vi "Average Sectors.vi"(11 "Preanalysis Stage":bool) -> ()   [LabVIEW 2013]
uses:
  Globals/Accumulated Sector Intensity.vi
  <vilib>/rvi/Memory/Memory_Emulation/nirvimemoryFastEmulationFpgaImpl.vi
  <instcachedir>/0/nirvimemoryFastEmulationFpgaImpl_5FBAB50466BC4C939F684F8805638BFC.lvgen/nirvimemoryFastEmulationFpgaImpl_5FBAB50466BC4C939F684F8805638BFC_001.vi
  <vilib>/rvi/DataTransferAndStorage/Container/Common/niFpgaContainerGetUniqueNameForEmu.vi
  <vilib>/rvi/Memory/Memory_Emulation/nirvimemoryFastEmulation.vi
  <vilib>/rvi/Memory/Memory_Emulation/nirvimemoryEmulation.vi
  Globals/Sector Parameter Global.vi
  <vilib>/rvi/FIFO/Fifo_Resource/nirvififoEmulationWriteFpgaImpl.vi
  <vilib>/rvi/DataTransferAndStorage/Container/XNode/niFpgaContainer.xnode
  <vilib>/rvi/FIFO/Fifo_Resource/nirvififoEmulationWrite.vi
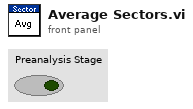
[diagram p1: front panel]
types:
  T1 = cluster{"Accumulated Intensity":fxp<+,20,20>, "Count":fxp<+,12,12>}[]
  T2 = cluster{"Accumulated Intensity":fxp<+,20,20>, "Count":fxp<+,12,12>}
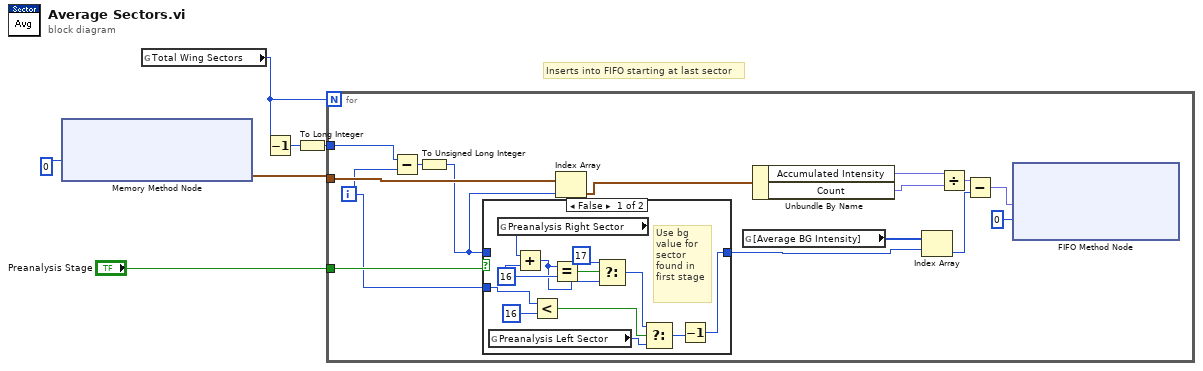
[diagram p0: block diagram]
diagram:
  # "Inserts into FIFO starting at last sector"
  n1 = xnode ("Memory Method Node")("Address"=u32 0) -> ("Data"=w2:T1)  [unwired: 1 in, 1 out]
  n2 = global read "Accumulated Sector Intensity.vi" "Total Wing Sectors"() -> (w4:u8)
  n3 = Decrement(x=w4) -> (x-1=w6:u8)
  n4 = To Long Integer(number=w6) -> (32bit integer=w5:i32)
  n5 = for {
    N: w4 -> [_]
    tunnel: w5 -> [w16]
    tunnel: w2 -> [w14]
    tunnel: "Preanalysis Stage" -> [w10]
    i -> [w7]
    n6 = Subtract(x=w16, y=w7) -> (x-y=w15:i32)
    n7 = To Unsigned Long Integer(number=w15) -> (unsigned 32bit integer=w8:u32)
    n8 = case shown="False" w10 {
      tunnel: [w28 w34] -> w9
      tunnel: w8 -> [_ w34]
      tunnel: w7 -> [w33 _]
      frame False {
        w26 = u8 16 ("y")
        # "Use bg value for sector found in first stage"
        n9 = global read "Sector Parameter Global.vi" "Preanalysis Left Sector"() -> (w30:u8)
        n10 = global read "Sector Parameter Global.vi" "Preanalysis Right Sector"() -> (w23:u8)
        n11 = Add(x=w23, y=w26) -> (x+y=w24:u8)
        n12 = Less?(x=w33, y=16) -> (x < y?=w31:bool)
        n13 = Equal?(x=w24, y=w26) -> (x = y?=w27:bool)
        n14 = Select(t=u8 17, s=w27, f=w24) -> (s? t:f=w22:u8)
        n15 = Select(t=w22, s=w31, f=w30) -> (s? t:f=w29:u8)
        n16 = Decrement(x=w29) -> (x-1=w28:u8)
      }
      frame True {
        # "For preanalysis, use the bg\nvalues for the 32 sectors"
      }
    }
    n17 = Index Array(array=w14, index=w8) -> (element=w13:T2)
    n18 = global read "Sector Parameter Global.vi" "[Average BG Intensity]"() -> (w20:u8[])
    n19 = Unbundle By Name(w13) -> ("Accumulated Intensity"=w12:fxp<+,20,20>, "Count"=w11:fxp<+,12,12>)
    n20 = Index Array(array=w20, index=w9) -> (element=w18:u8)
    n21 = Divide(x=w12, y=w11) -> (x/y=w19:fxp<+,8,8>)
    n22 = Subtract(x=w19, y=w18) -> (x-y=w17:fxp<+/-,9,9>)
    n23 = xnode ("FIFO Method Node")("Element"=w17, "Timeout"=0) -> ()  [unwired: 1 in, 2 out]
  }
